vi "Pad.vi"(0 "Message Length (bytes)":i32, 11 "Last Part":u8[](array[numeric])) -> (8 "Padding":u8[](array[numeric]) format="%.0x")   [LabVIEW 2020, in "Crypto.lvlib" / "SHA-1.lvclass"]
uses:
  SHA-1.lvclass
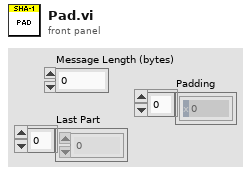
[diagram p1: front panel]
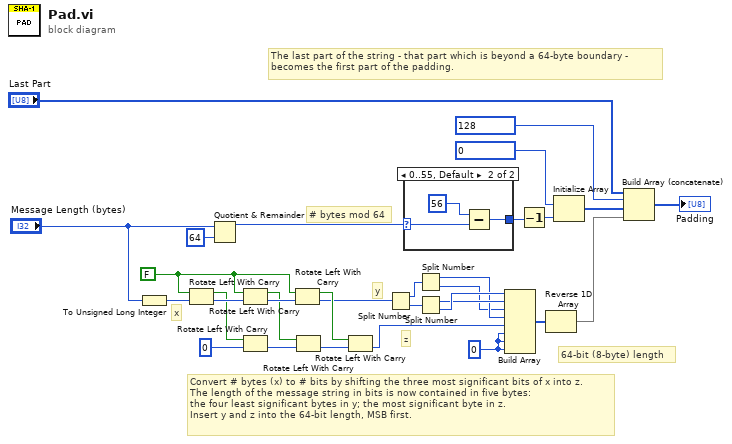
[diagram p0: block diagram]
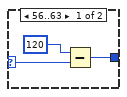
[diagram p2: hidden frame]
diagram:
  w19 = FALSE ("carry")
  w22 = u8 0
  # "The last part of the string - that part which is beyond a 64-byte boundary -\nbecomes the first part of the padding."
  # "64-bit (8-byte) length"
  # "x"
  # "y"
  # "z"
  # "Convert # bytes (x) to # bits by shifting the three most significant bits of x into z.\nThe length of the message string in bits is now contained in five bytes:  \nthe four least significant bytes in y; the most significant byte in z.\nInsert y and z into the 64-bit length, MSB first."
  # "# bytes mod 64"
  n1 = To Unsigned Long Integer(number="Message Length (bytes)") -> (unsigned 32bit integer=w8:u32)
  n2 = Rotate Left With Carry(2:w8, 3:w19) -> (0:w20:u32, 1:w16:bool)
  n3 = Quotient & Remainder(x="Message Length (bytes)", y=64) -> (x-y*floor(x/y)=w7:i32)  [unwired: 1 out]
  n4 = Rotate Left With Carry(2:w20, 3:w19) -> (0:w18:u32, 1:w14:bool)
  n5 = Rotate Left With Carry(2:u8 0, 3:w16) -> (0:w15:u8)  [unwired: 1 out]
  n6 = Rotate Left With Carry(2:w18, 3:w19) -> (0:w11:u32, 1:w12:bool)
  n7 = Rotate Left With Carry(2:w15, 3:w14) -> (0:w13:u8)  [unwired: 1 out]
  n8 = Rotate Left With Carry(2:w13, 3:w12) -> (0:w10:u8)  [unwired: 1 out]
  n9 = Split Number(x=w11) -> (hi(x)=w27:u16, lo(x)=w26:u16)
  n10 = case shown="0..55, Default" w7 {
    selector: w7 -> [w33 w36]
    tunnel: [w32 w35] -> w9
    frame 56..63 {
      n11 = Subtract(x=i64 120, y=w33) -> (x-y=w32:i64)
    }
    frame 0..55, Default {
      n12 = Subtract(x=i64 56, y=w36) -> (x-y=w35:i64)
    }
  }
  n13 = Split Number(x=w27) -> (hi(x)=w23:u8, lo(x)=w6:u8)
  n14 = Split Number(x=w26) -> (hi(x)=w24:u8, lo(x)=w25:u8)
  n15 = Build Array(w25, w24, w6, w23, w10, w22, w22, w22) -> (w4:u8[])
  n16 = Decrement(x=w9) -> (x-1=w21:i64)
  n17 = Reverse 1D Array(array=w4) -> (reversed array=w3:u8[])
  n18 = Initialize Array(u8 0, w21) -> (w30:u8[])
  n19 = Build Array (concatenate)("Last Part", u8 128, w30, w3) -> (→"Padding":u8[])
